vi "ZPL GEN Convert Errors.vi"(8 "error":errorcluster, 9 "Expect \"OK\" (F)":bool=TRUE, 10 "String in":string, 11 "VISA":refnum<visa-resource-name>="COM1") -> (0 "error out":errorcluster={"status"=TRUE, "code"=-1074001403, "source"="<Err>Setting out of range.  Attempt to program a setting outside of the model rating."}, 3 "VISA out":refnum<visa-resource-name>)   [LabVIEW 2016]
doc: "This vi inputs a string and compares it to all possible Genesys error messages (ex: \"C01\" or \"E04\"). If the response is in the error list, a VISA error number is assigned to it and the error description is passed out the \"error out\" cluster.\n\nIf \"Expect \"OK\"\" is set TRUE, a special error will be passed if the response is not not in the error list and if it is not \"OK\""
panel:
  in  "Error List":T1(array[cluster])=[{"String"="E01", "Code"=-1074001663, "Descr"="<Err>Attemp to set the voltage setting too high. Conflicts with the over-voltage protection."}, {"String"="E02", "Code"=-1074001662, "Descr"="<Err>Attemp to set the voltage setting too low. Conflicts with the under-voltage limit."}, {"String"="E04", "Code"=-1074001660, "Descr"="<Err>Attemp to set the over-voltage protection  too low.  Conflicts with the voltage setting."}, {"String"="E06", "Code"=-1074001658, "Descr"="<Err>Attempt to set the under-voltage limit too high.  Conflicts with the voltage setting."}, {"String"="E07", "Code"=-1074001657, "Descr"="<Err>Attempt to turn the output ON while a fault is keeping the output OFF."}, {"String"="E08", "Code"=-1074001656, "Descr"="<Err>Attempt to send command to power supply in ADSL mode"}, {"String"="C01", "Code"=-1074001407, "Descr"="<Err>Illegal command or query."}, {"String"="C02", "Code"=-1074001406, "Descr"="<Err>Missing parameter.  Command requires a value but the value is missing."}, {"String"="C03", "Code"=-1074001405, "Descr"="<Err>Illegal parameter.  Command requires a value but value is wrong type."}, {"String"="C04", "Code"=-1074001404, "Descr"="<Err>Checksum error.  Genesys received message with checksum but the checksum did not verify correctly."}, {"String"="C05", "Code"=-1074001403, "Descr"="<Err>Setting out of range.  Attempt to program a setting outside of the model rating."}]
  # "Convert Errors"
  # "Lambda ZPLUS \n Serial Port\n  DC Power Supplies"
  # "Match input string to list of\n    Genesys error messages.\nConvert error message to \n    VISA error code."
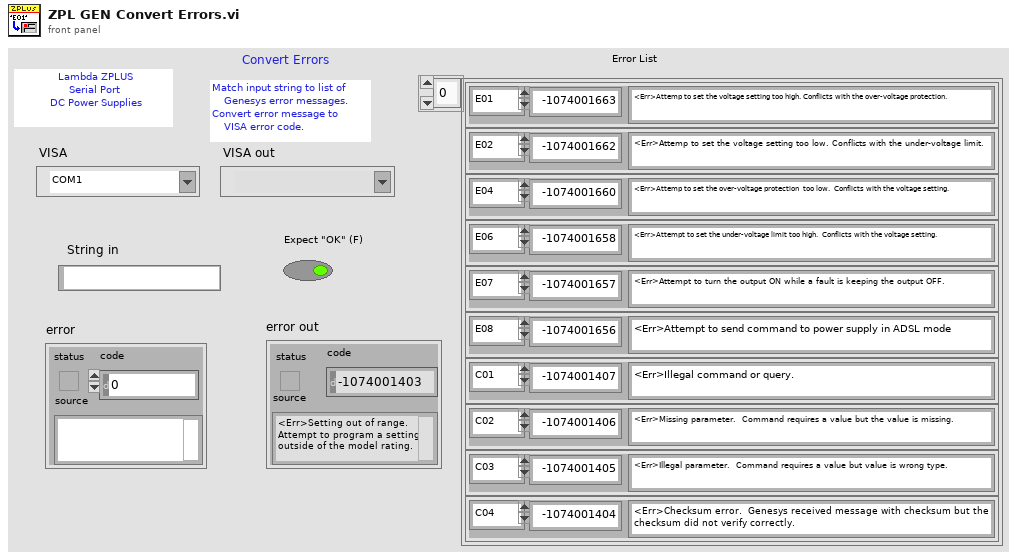
[diagram p1: front panel]
types:
  T1 = cluster{"String":string, "Code":i32, "Descr":string}[]
  T2 = cluster{"String":string, "Code":i32, "Descr":string}
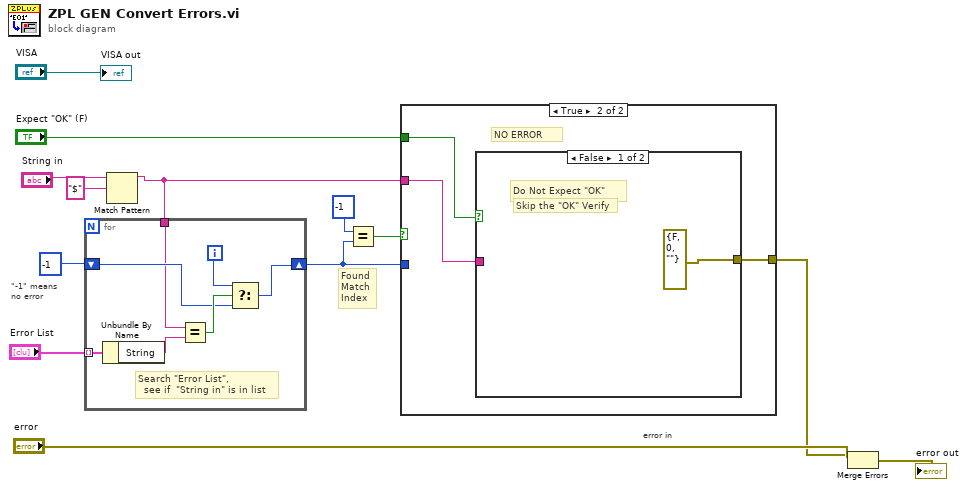
[diagram p0: block diagram]
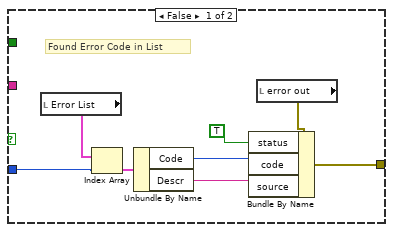
[diagram p2: hidden frame]
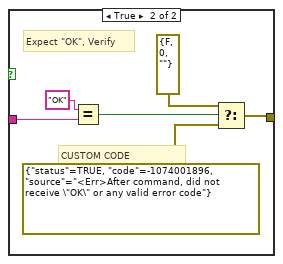
[diagram p3: hidden frame]
diagram:
  # "error in"
  # "Found\nMatch\nIndex"
  # "\"-1\" means\nno error"
  n1 = Match Pattern(string="String in", regular expression="$") -> (before substring=w1:string)  [unwired: 1 in, 3 out]
  n2 = for {
    tunnel: "Error List" -> [w18] mode=indexing
    shift-right: [w15] -> w9
    shift-left: -1 -> [w16]
    tunnel: w1 -> [w14]
    i -> [w17]
    # "Search \"Error List\", \n  see if  \"String in\" is in list"
    n3 = Unbundle By Name(w18) -> ("String"=w20:string)
    n4 = Equal?(x=w14, y=w20) -> (x = y?=w19:bool)
    n5 = Select(t=w17, s=w19, f=w16) -> (s? t:f=w15:i32)
  }
  n6 = Equal?(x=-1, y=w9) -> (x = y?=w10:bool)
  n7 = case shown="True" w10 {
    tunnel: w9 -> [w26 _]
    tunnel: [w22 w30] -> w6
    tunnel: w1 -> [_ w31]
    tunnel: "Expect \"OK\" (F)" -> [_ w29]
    frame False {
      # "Found Error Code in List"
      n8 = local read "Error List"() -> (w27:T1)
      n9 = Index Array(array=w27, index=w26) -> (element=w25:T2)
      n10 = Unbundle By Name(w25) -> ("Code"=w24:i32, "Descr"=w21:string)
      n11 = local read "error out"() -> (w28:errorcluster)
      n12 = Bundle By Name(cluster=w28, "status"=TRUE, "code"=w24, "source"=w21) -> (w22:errorcluster)
    }
    frame True {
      # "NO ERROR"
      n13 = case shown="False" w29 {
        tunnel: w31 -> [_ w34]
        tunnel: [errorcluster {"status"=FALSE, "code"=0, "source"=""} ("error") w36] -> w30
        frame False {
          # "Skip the \"OK\" Verify"
          # "Do Not Expect \"OK\""
        }
        frame True {
          # "CUSTOM CODE"
          # "Expect \"OK\", Verify"
          n14 = Equal?(x="OK", y=w34) -> (x = y?=w33:bool)
          n15 = Select(t=errorcluster {"status"=FALSE, "code"=0, "source"=""} ("error"), s=w33, f=errorcluster {"status"=TRUE, "code"=-1074001896, "source"="<Err>After command, did not receive \"OK\" or any valid error code"} ("error")) -> (s? t:f=w36:errorcluster)
        }
      }
    }
  }
  n16 = Merge Errors("error", w6) -> (→"error out":errorcluster)
  "VISA out" <- "VISA"
